vi "Subvi counter up U64.vi"(4 "Reset":bool, 6 "Gating":bool, 8 "Trigger":bool) -> (1 "Output":u64)   [LabVIEW 2017]
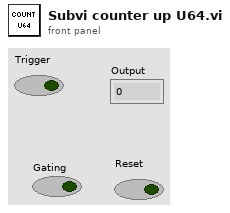
[diagram p1: front panel]
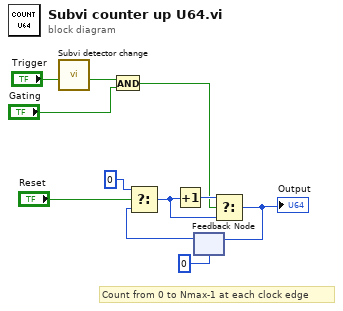
[diagram p0: block diagram]
diagram:
  # "Count from 0 to Nmax-1 at each clock edge"
  n1 = call "Subvi detector change.vi"("Input"="Trigger") -> ("Output"=w4:bool)  [unwired: 8 in]
  n2 = And(x=w4, y="Gating") -> (x .and. y?=w2:bool)
  n3 = feedback #1(u64 0) -> (w6:u64)
  n4 = Select(t=u64 0, s="Reset", f=w6) -> (s? t:f=w7:u64)
  n5 = Increment(x=w7) -> (x+1=w8:u64)
  n6 = Select(t=w8, s=w2, f=w7) -> (s? t:f=w10:u64)
  "Output" <- w10
  n7 = feedback-in #1(w10) -> ()
